vi "关键参数交互.vi"(9 "量程下拉列表":refnum<vi>, 10 "测量模式下拉列表":refnum<vi>, 11 "参数下拉列表":refnum<vi>) -> ()   [LabVIEW 2016, in "斯坦道总磷总氮.lvlib"]
panel:
  out "x != y? 4":T1
  out "x != y? 3":T1
  out "x != y? 2":T1
  out "x != y?":T1
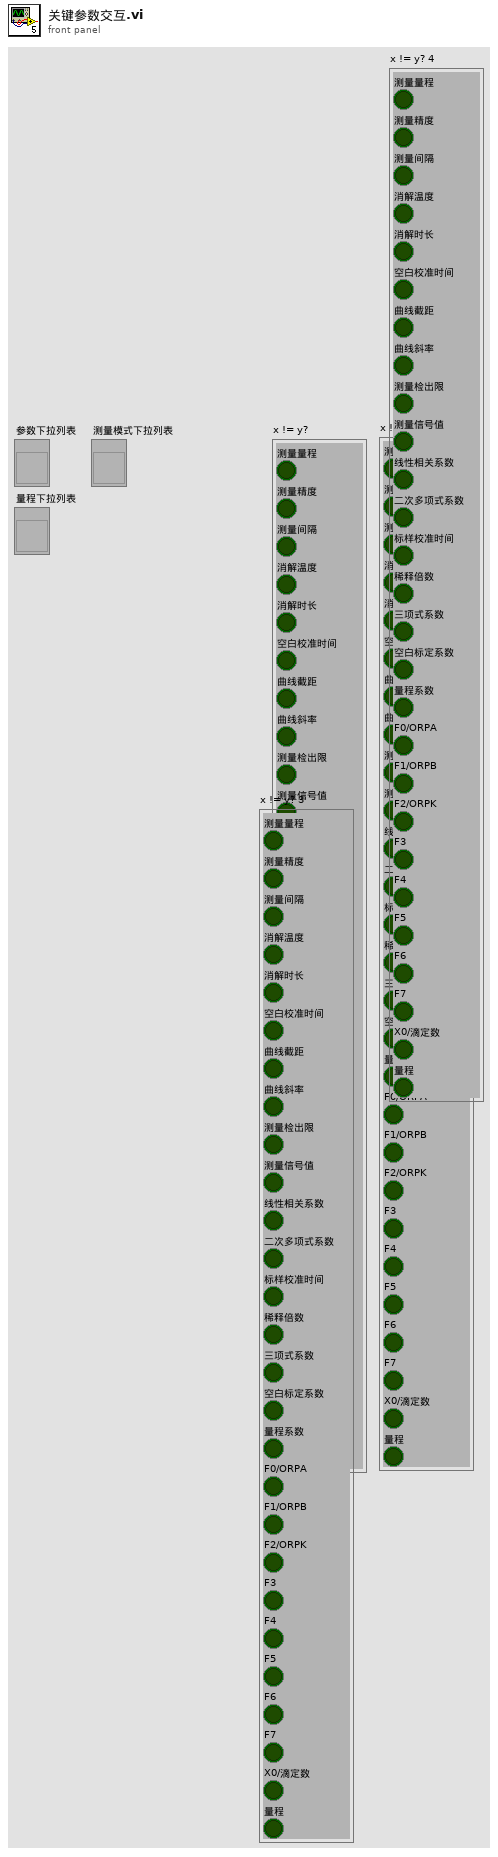
[diagram p1: front panel]
types:
  T1 = cluster{"测量量程":bool, "测量精度":bool, "测量间隔":bool, "消解温度":bool, "消解时长":bool, "空白校准时间":bool, "曲线截距":bool, "曲线斜率":bool, "测量检出限":bool, "测量信号值":bool, "线性相关系数":bool, "二次多项式系数":bool, "标样校准时间":bool, "稀释倍数":bool, "三项式系数":bool, "空白标定系数":bool, "量程系数":bool, "F0/ORPA":bool, "F1/ORPB":bool, "F2/ORPK":bool, "F3":bool, "F4":bool, "F5":bool, "F6":bool, "F7":bool, "X0/滴定数":bool, "量程":bool}
  T2 = cluster{"COD":bool, "氨氮":bool, "总氮":bool, "总磷":bool}
  T3 = cluster{"测量量程":dbl, "测量精度":dbl, "测量间隔":dbl, "消解温度":dbl, "消解时长":dbl, "空白校准时间":timestamp, "曲线截距":dbl, "曲线斜率":dbl, "测量检出限":dbl, "测量信号值":dbl, "线性相关系数":dbl, "二次多项式系数":dbl, "标样校准时间":timestamp, "稀释倍数":dbl, "三项式系数":dbl, "空白标定系数":dbl, "量程系数":dbl, "F0/ORPA":dbl, "F1/ORPB":dbl, "F2/ORPK":dbl, "F3":dbl, "F4":dbl, "F5":dbl, "F6":dbl, "F7":dbl, "X0/滴定数":dbl, "量程":dbl}
  T4 = cluster{"chose":string, "公式":cluster{"X^2":dbl, "X":dbl, "b":dbl}}
  T5 = cluster{"时间标识":timestamp, "设备":string, "日志信息":string, "流程参数":string}
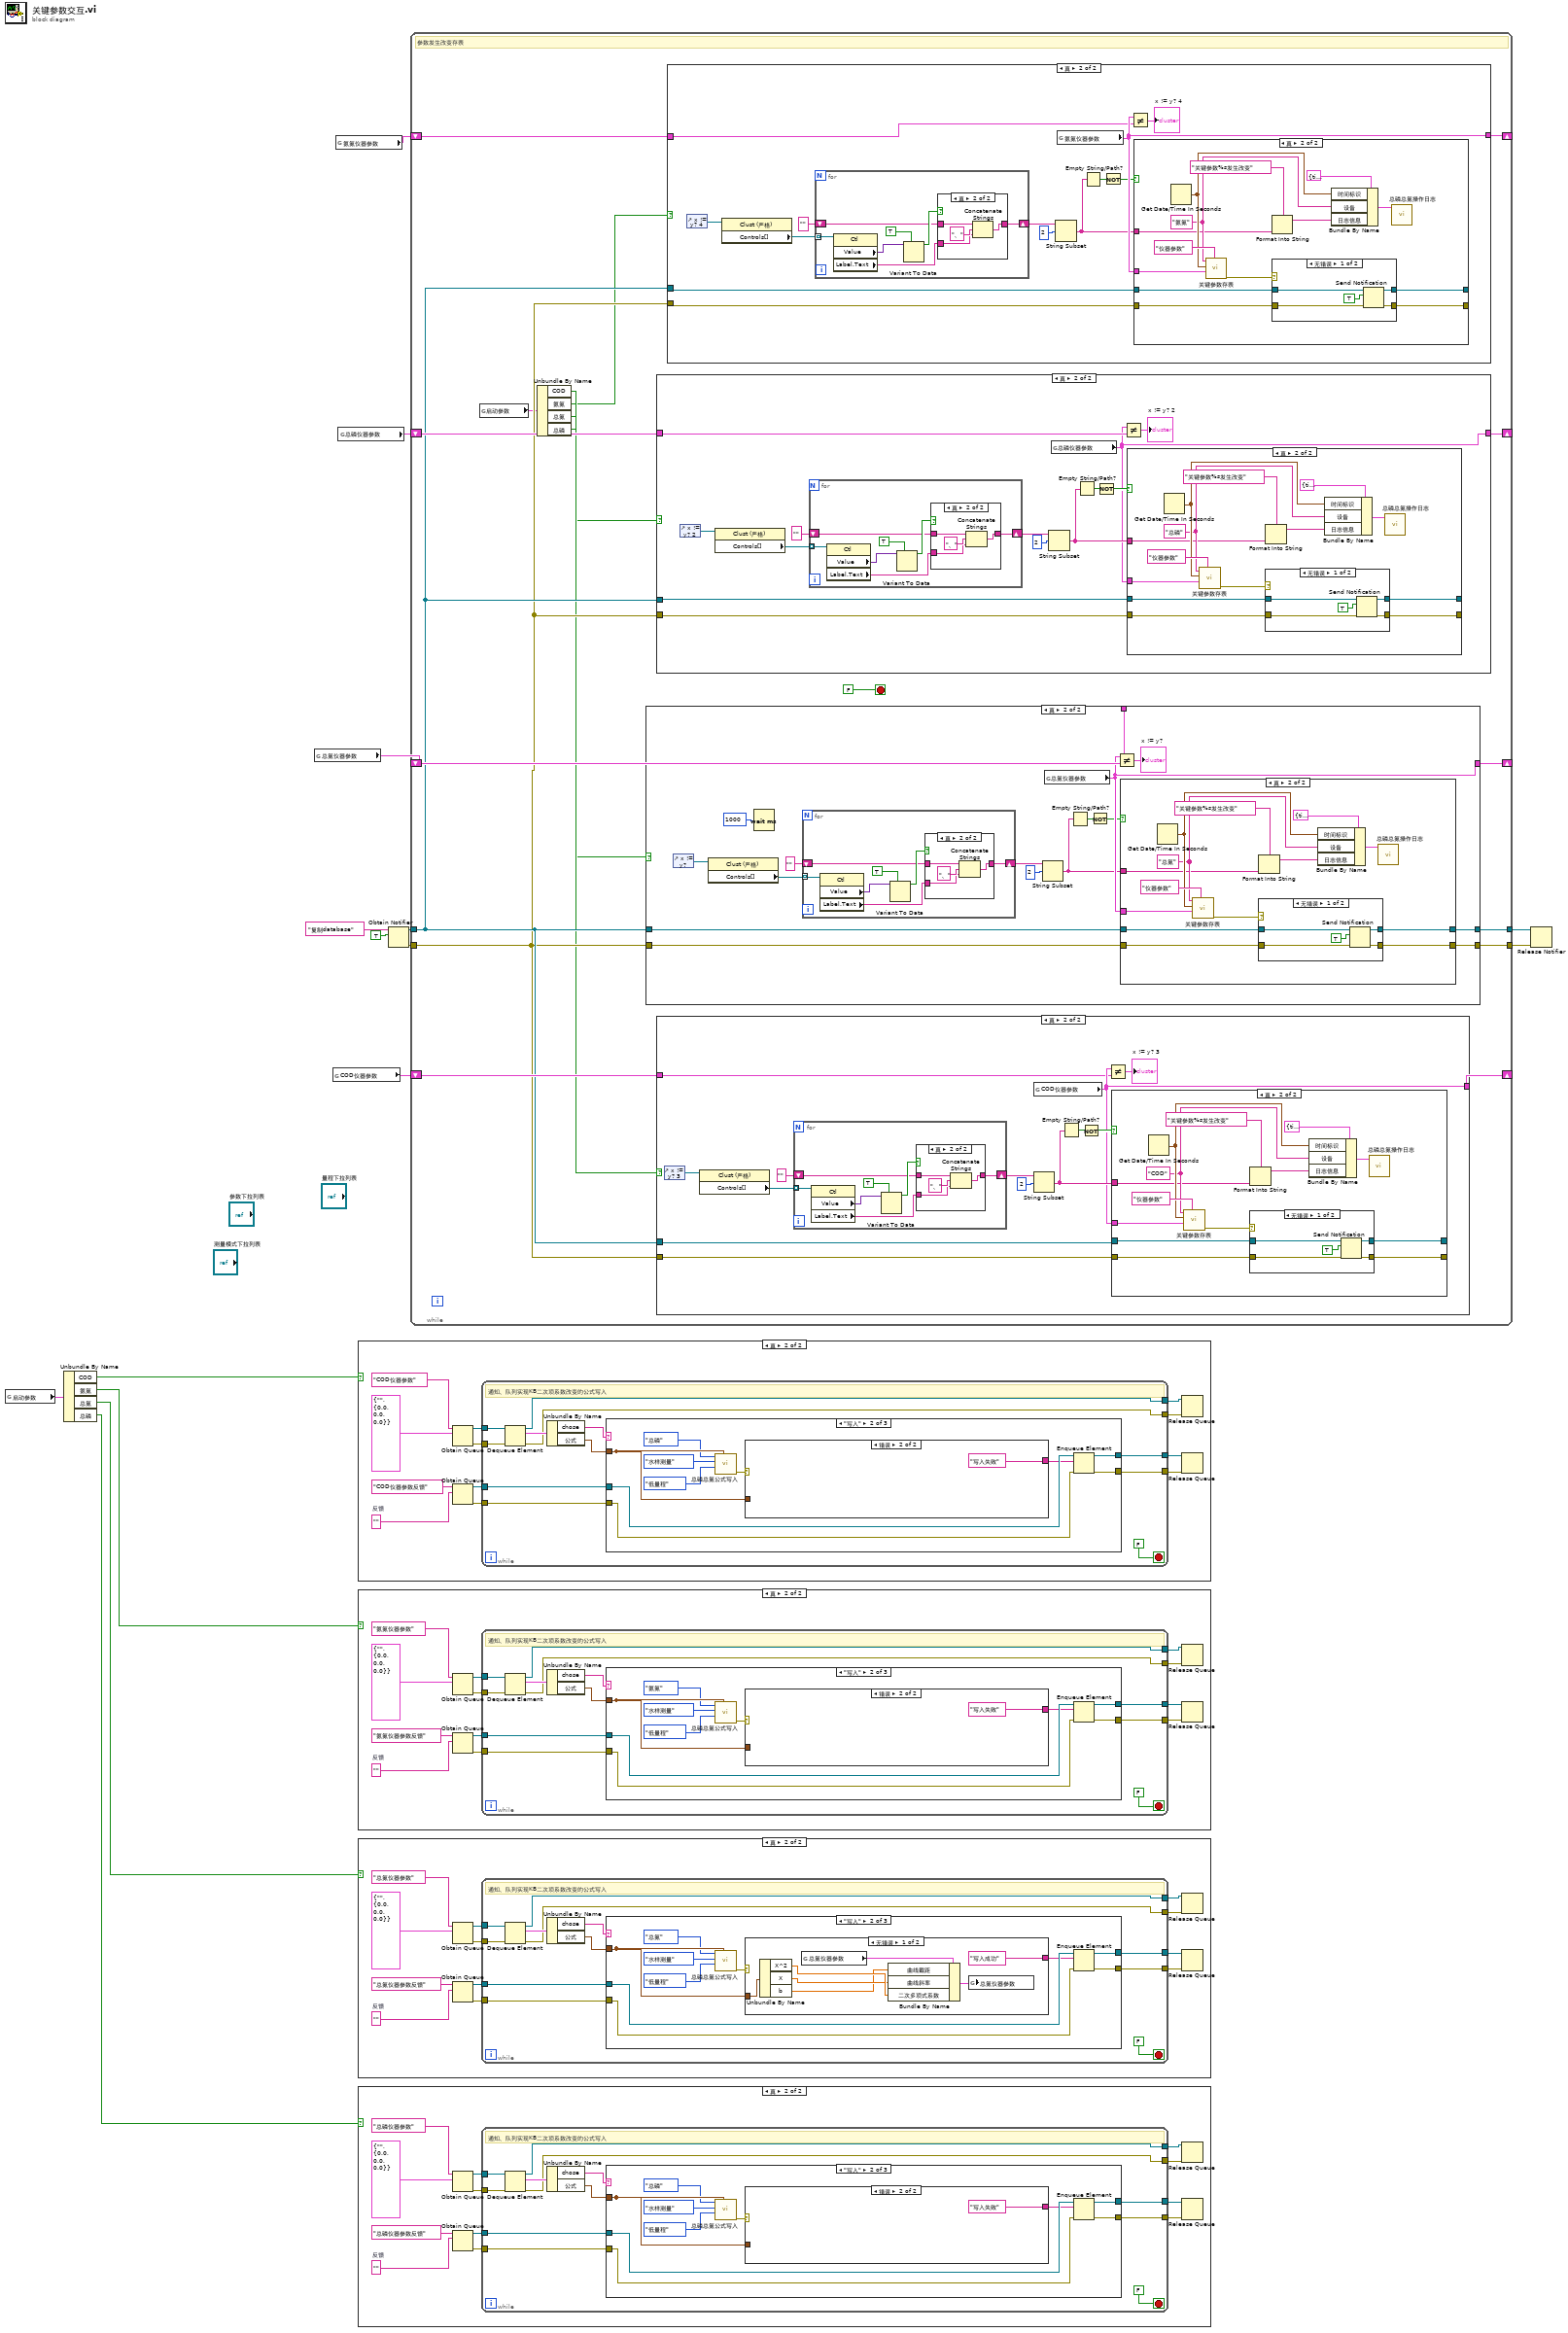
[diagram p0: block diagram]
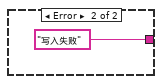
[diagram p4: hidden frame]
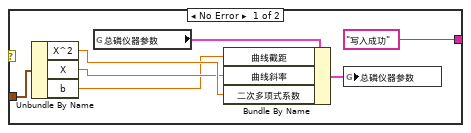
[diagram p8: hidden frame]
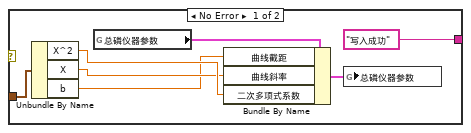
[diagram p12: hidden frame]
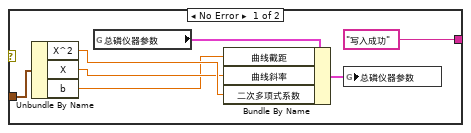
[diagram p16: hidden frame]
diagram:
  n1 = global read "总磷总氮断电保存全局变量.vi" "启动参数"() -> (w6:T2)
  n2 = Unbundle By Name(w6) -> ("COD"=w5:bool, "氨氮"=w4:bool, "总氮"=w2:bool, "总磷"=w3:bool)
  n3 = global read "总磷总氮断电保存全局变量.vi" "总氮仪器参数"() -> (w15:T3)
  n4 = global read "总磷总氮断电保存全局变量.vi" "COD仪器参数"() -> (w7:T3)
  n5 = global read "总磷总氮断电保存全局变量.vi" "氨氮仪器参数"() -> (w1:T3)
  n6 = global read "总磷总氮断电保存全局变量.vi" "总磷仪器参数"() -> (w8:T3)
  n7 = case shown="真" w5 {
    frame False {
    }
    frame True {
      w22 = ""  # 反馈
      n8 = Obtain Queue(name (unnamed)="COD仪器参数" ("名称（未命名）"), element data type=T4 {"chose"="", "公式"={"X^2"=0.0, "X"=0.0, "b"=0.0}}) -> (queue out=w26:refnum<queue>, error out=w27:errorcluster)  [unwired: 3 in, 1 out]
      n9 = Obtain Queue(name (unnamed)="COD仪器参数反馈" ("名称（未命名）"), element data type=w22) -> (queue out=w21:refnum<queue>, error out=w23:errorcluster)  [unwired: 3 in, 1 out]
      n10 = while {
        tunnel: w26 -> [w38]
        tunnel: w27 -> [w37]
        tunnel: [w29] -> w18
        tunnel: [w28] -> w19
        tunnel: w21 -> [w33]
        tunnel: w23 -> [w32]
        tunnel: [w31] -> w24
        tunnel: [w30] -> w25
        stop <- FALSE stop-if-true
        # "通知、队列实现KB二次项系数改变的公式写入"
        n11 = Dequeue Element(queue=w38, error in (no error)=w37) -> (queue out=w29:refnum<queue>, element=w36:T4, error out=w28:errorcluster)  [unwired: 1 in, 1 out]
        n12 = Unbundle By Name(w36) -> ("chose"=w35:string, "公式"=w34:cluster{"X^2":dbl, "X":dbl, "b":dbl})
        n13 = case shown="\"写入\"" w35 {
          tunnel: w34 -> [_ w45 _]
          tunnel: w33 -> [w41 w50 w61]
          tunnel: w32 -> [w40 w48 w60]
          tunnel: [w41 w47 w61] -> w31
          tunnel: [w40 w46 w60] -> w30
          frame "假", Default {
          }
          frame "写入" {
            n14 = call "总磷总氮公式写入.vi"("公式"=w45, "量程"=enum16{"低量程", "高量程"}."低量程", "测量模式"=enum16{"水样测量", "零点核查", "跨度核查", "标样核查", "加标回收"}."水样测量", "测量参数"=enum16{"COD", "氨氮", "总氮", "总磷"}."总磷") -> ("error out"=w51:errorcluster)  [unwired: 7 in]
            n15 = case shown="错误" w51 {
              tunnel: ["写入成功" ("消息") "写入失败" ("消息")] -> w49
              tunnel: w45 -> [w55 _]
              frame No Error {
                n16 = Unbundle By Name(w55) -> ("X^2"=w54:dbl, "X"=w53:dbl, "b"=w52:dbl)
                n17 = global read "总磷总氮断电保存全局变量.vi" "总磷仪器参数"() -> (w56:T3)
                n18 = Bundle By Name(cluster=w56, "曲线截距"=w52, "曲线斜率"=w53, "二次多项式系数"=w54) -> (w57:T3)
                n19 = global write "总磷总氮断电保存全局变量.vi" "总磷仪器参数"(w57) -> ()
              }
              frame Error {
              }
            }
            n20 = Enqueue Element(queue=w50, element=w49, error in (no error)=w48) -> (queue out=w47:refnum<queue>, error out=w46:errorcluster)  [unwired: 1 in, 1 out]
          }
          frame "读取" {
          }
        }
      }
      n21 = Release Queue(queue=w18, error in (no error)=w19) -> ()  [unwired: 1 in, 3 out]
      n22 = Release Queue(queue=w24, error in (no error)=w25) -> ()  [unwired: 1 in, 3 out]
    }
  }
  n23 = case shown="真" w4 {
    frame False {
    }
    frame True {
      w67 = ""  # 反馈
      n24 = Obtain Queue(name (unnamed)="氨氮仪器参数" ("名称（未命名）"), element data type=T4 {"chose"="", "公式"={"X^2"=0.0, "X"=0.0, "b"=0.0}}) -> (queue out=w63:refnum<queue>, error out=w62:errorcluster)  [unwired: 3 in, 1 out]
      n25 = Obtain Queue(name (unnamed)="氨氮仪器参数反馈" ("名称（未命名）"), element data type=w67) -> (queue out=w68:refnum<queue>, error out=w66:errorcluster)  [unwired: 3 in, 1 out]
      n26 = while {
        tunnel: w63 -> [w84]
        tunnel: w62 -> [w83]
        tunnel: [w75] -> w71
        tunnel: [w74] -> w70
        tunnel: w68 -> [w79]
        tunnel: w66 -> [w78]
        tunnel: [w77] -> w65
        tunnel: [w76] -> w64
        stop <- FALSE stop-if-true
        # "通知、队列实现KB二次项系数改变的公式写入"
        n27 = Dequeue Element(queue=w84, error in (no error)=w83) -> (queue out=w75:refnum<queue>, element=w82:T4, error out=w74:errorcluster)  [unwired: 1 in, 1 out]
        n28 = Unbundle By Name(w82) -> ("chose"=w81:string, "公式"=w80:cluster{"X^2":dbl, "X":dbl, "b":dbl})
        n29 = case shown="\"写入\"" w81 {
          tunnel: w80 -> [_ w91 _]
          tunnel: w79 -> [w87 w96 w107]
          tunnel: w78 -> [w86 w94 w106]
          tunnel: [w87 w93 w107] -> w77
          tunnel: [w86 w92 w106] -> w76
          frame "假", Default {
          }
          frame "写入" {
            n30 = call "总磷总氮公式写入.vi"("公式"=w91, "量程"=enum16{"低量程", "高量程"}."低量程", "测量模式"=enum16{"水样测量", "零点核查", "跨度核查", "标样核查", "加标回收"}."水样测量", "测量参数"=enum16{"COD", "氨氮", "总氮", "总磷"}."氨氮") -> ("error out"=w97:errorcluster)  [unwired: 7 in]
            n31 = case shown="错误" w97 {
              tunnel: ["写入成功" ("消息") "写入失败" ("消息")] -> w95
              tunnel: w91 -> [w101 _]
              frame No Error {
                n32 = Unbundle By Name(w101) -> ("X^2"=w100:dbl, "X"=w99:dbl, "b"=w98:dbl)
                n33 = global read "总磷总氮断电保存全局变量.vi" "总磷仪器参数"() -> (w102:T3)
                n34 = Bundle By Name(cluster=w102, "曲线截距"=w98, "曲线斜率"=w99, "二次多项式系数"=w100) -> (w103:T3)
                n35 = global write "总磷总氮断电保存全局变量.vi" "总磷仪器参数"(w103) -> ()
              }
              frame Error {
              }
            }
            n36 = Enqueue Element(queue=w96, element=w95, error in (no error)=w94) -> (queue out=w93:refnum<queue>, error out=w92:errorcluster)  [unwired: 1 in, 1 out]
          }
          frame "读取" {
          }
        }
      }
      n37 = Release Queue(queue=w71, error in (no error)=w70) -> ()  [unwired: 1 in, 3 out]
      n38 = Release Queue(queue=w65, error in (no error)=w64) -> ()  [unwired: 1 in, 3 out]
    }
  }
  n39 = case shown="真" w2 {
    frame False {
    }
    frame True {
      w113 = ""  # 反馈
      n40 = Obtain Queue(name (unnamed)="总氮仪器参数" ("名称（未命名）"), element data type=T4 {"chose"="", "公式"={"X^2"=0.0, "X"=0.0, "b"=0.0}}) -> (queue out=w109:refnum<queue>, error out=w108:errorcluster)  [unwired: 3 in, 1 out]
      n41 = Obtain Queue(name (unnamed)="总氮仪器参数反馈" ("名称（未命名）"), element data type=w113) -> (queue out=w114:refnum<queue>, error out=w112:errorcluster)  [unwired: 3 in, 1 out]
      n42 = while {
        tunnel: w109 -> [w130]
        tunnel: w108 -> [w129]
        tunnel: [w121] -> w117
        tunnel: [w120] -> w116
        tunnel: w114 -> [w125]
        tunnel: w112 -> [w124]
        tunnel: [w123] -> w111
        tunnel: [w122] -> w110
        stop <- FALSE stop-if-true
        # "通知、队列实现KB二次项系数改变的公式写入"
        n43 = Dequeue Element(queue=w130, error in (no error)=w129) -> (queue out=w121:refnum<queue>, element=w128:T4, error out=w120:errorcluster)  [unwired: 1 in, 1 out]
        n44 = Unbundle By Name(w128) -> ("chose"=w127:string, "公式"=w126:cluster{"X^2":dbl, "X":dbl, "b":dbl})
        n45 = case shown="\"写入\"" w127 {
          tunnel: w126 -> [_ w137 _]
          tunnel: w125 -> [w133 w142 w153]
          tunnel: w124 -> [w132 w140 w152]
          tunnel: [w133 w139 w153] -> w123
          tunnel: [w132 w138 w152] -> w122
          frame "假", Default {
          }
          frame "写入" {
            n46 = call "总磷总氮公式写入.vi"("公式"=w137, "量程"=enum16{"低量程", "高量程"}."低量程", "测量模式"=enum16{"水样测量", "零点核查", "跨度核查", "标样核查", "加标回收"}."水样测量", "测量参数"=enum16{"COD", "氨氮", "总氮", "总磷"}."总氮") -> ("error out"=w143:errorcluster)  [unwired: 7 in]
            n47 = case shown="无错误" w143 {
              tunnel: ["写入成功" ("消息") "写入失败" ("消息")] -> w141
              tunnel: w137 -> [w147 _]
              frame No Error {
                n48 = Unbundle By Name(w147) -> ("X^2"=w146:dbl, "X"=w145:dbl, "b"=w144:dbl)
                n49 = global read "总磷总氮断电保存全局变量.vi" "总氮仪器参数"() -> (w148:T3)
                n50 = Bundle By Name(cluster=w148, "曲线截距"=w144, "曲线斜率"=w145, "二次多项式系数"=w146) -> (w149:T3)
                n51 = global write "总磷总氮断电保存全局变量.vi" "总氮仪器参数"(w149) -> ()
              }
              frame Error {
              }
            }
            n52 = Enqueue Element(queue=w142, element=w141, error in (no error)=w140) -> (queue out=w139:refnum<queue>, error out=w138:errorcluster)  [unwired: 1 in, 1 out]
          }
          frame "读取" {
          }
        }
      }
      n53 = Release Queue(queue=w117, error in (no error)=w116) -> ()  [unwired: 1 in, 3 out]
      n54 = Release Queue(queue=w111, error in (no error)=w110) -> ()  [unwired: 1 in, 3 out]
    }
  }
  n55 = case shown="真" w3 {
    frame False {
    }
    frame True {
      w160 = ""  # 反馈
      n56 = Obtain Queue(name (unnamed)="总磷仪器参数" ("名称（未命名）"), element data type=T4 {"chose"="", "公式"={"X^2"=0.0, "X"=0.0, "b"=0.0}}) -> (queue out=w164:refnum<queue>, error out=w165:errorcluster)  [unwired: 3 in, 1 out]
      n57 = Obtain Queue(name (unnamed)="总磷仪器参数反馈" ("名称（未命名）"), element data type=w160) -> (queue out=w159:refnum<queue>, error out=w161:errorcluster)  [unwired: 3 in, 1 out]
      n58 = while {
        tunnel: w164 -> [w176]
        tunnel: w165 -> [w175]
        tunnel: [w167] -> w156
        tunnel: [w166] -> w157
        tunnel: w159 -> [w171]
        tunnel: w161 -> [w170]
        tunnel: [w169] -> w162
        tunnel: [w168] -> w163
        stop <- FALSE stop-if-true
        # "通知、队列实现KB二次项系数改变的公式写入"
        n59 = Dequeue Element(queue=w176, error in (no error)=w175) -> (queue out=w167:refnum<queue>, element=w174:T4, error out=w166:errorcluster)  [unwired: 1 in, 1 out]
        n60 = Unbundle By Name(w174) -> ("chose"=w173:string, "公式"=w172:cluster{"X^2":dbl, "X":dbl, "b":dbl})
        n61 = case shown="\"写入\"" w173 {
          tunnel: w172 -> [_ w183 _]
          tunnel: w171 -> [w179 w188 w199]
          tunnel: w170 -> [w178 w186 w198]
          tunnel: [w179 w185 w199] -> w169
          tunnel: [w178 w184 w198] -> w168
          frame "假", Default {
          }
          frame "写入" {
            n62 = call "总磷总氮公式写入.vi"("公式"=w183, "量程"=enum16{"低量程", "高量程"}."低量程", "测量模式"=enum16{"水样测量", "零点核查", "跨度核查", "标样核查", "加标回收"}."水样测量", "测量参数"=enum16{"COD", "氨氮", "总氮", "总磷"}."总磷") -> ("error out"=w189:errorcluster)  [unwired: 7 in]
            n63 = case shown="错误" w189 {
              tunnel: ["写入成功" ("消息") "写入失败" ("消息")] -> w187
              tunnel: w183 -> [w193 _]
              frame No Error {
                n64 = Unbundle By Name(w193) -> ("X^2"=w192:dbl, "X"=w191:dbl, "b"=w190:dbl)
                n65 = global read "总磷总氮断电保存全局变量.vi" "总磷仪器参数"() -> (w194:T3)
                n66 = Bundle By Name(cluster=w194, "曲线截距"=w190, "曲线斜率"=w191, "二次多项式系数"=w192) -> (w195:T3)
                n67 = global write "总磷总氮断电保存全局变量.vi" "总磷仪器参数"(w195) -> ()
              }
              frame Error {
              }
            }
            n68 = Enqueue Element(queue=w188, element=w187, error in (no error)=w186) -> (queue out=w185:refnum<queue>, error out=w184:errorcluster)  [unwired: 1 in, 1 out]
          }
          frame "读取" {
          }
        }
      }
      n69 = Release Queue(queue=w156, error in (no error)=w157) -> ()  [unwired: 1 in, 3 out]
      n70 = Release Queue(queue=w162, error in (no error)=w163) -> ()  [unwired: 1 in, 3 out]
    }
  }
  n71 = Obtain Notifier(name (unnamed)="复制database" ("名称（未命名）"), notification data type=TRUE) -> (notifier out=w12:refnum<notifier>, error out=w11:errorcluster)  [unwired: 2 in, 1 out]
  n72 = while {
    shift-right: [w216] -> _
    shift-left: w15 -> [w217]
    tunnel: w12 -> [w207]
    tunnel: w11 -> [w206]
    tunnel: [w215] -> w10
    tunnel: [w214] -> w9
    shift-right: [w212] -> _
    shift-left: w8 -> [w213]
    shift-right: [w211] -> _
    shift-left: w7 -> [w210]
    shift-right: [w209] -> _
    shift-left: w1 -> [w208]
    stop <- FALSE stop-if-true
    # "参数发生改变存表"
    n73 = global read "总磷总氮断电保存全局变量.vi" "启动参数"() -> (w204:T2)
    n74 = Unbundle By Name(w204) -> ("COD"=w203:bool, "氨氮"=w200:bool, "总氮"=w202:bool, "总磷"=w201:bool)
    n75 = case shown="真" w202 {
      tunnel: w217 -> [w269 w284]
      tunnel: [w269 w281] -> w216
      tunnel: [w268 w280] -> w215
      tunnel: [w267 w279] -> w214
      tunnel: w207 -> [w268 w271]
      tunnel: w206 -> [w267 w270]
      frame False {
      }
      frame True {
        n76 = control-ref of="x != y?"() -> (w282:refnum<vi>)
        n77 = property class="Clust (严格)"(reference=w282) -> ("Controls[]"=w275:refnum<vi>[])  [unwired: 1 in, 2 out]
        n78 = Wait (ms)(milliseconds to wait=u32 1000 ("等待时间（毫秒）")) -> ()  [unwired: 1 out]
        n79 = for {
          tunnel: w275 -> [w292] mode=indexing
          shift-right: [w286] -> w277
          shift-left: "" -> [w288]
          n80 = property class="Ctl"(reference=w292) -> ("Value"=w290:variant, "Label.Text"=w287:string)  [unwired: 1 in, 2 out]
          n81 = Variant To Data(type=TRUE, Variant=w290) -> (data=w289:bool)  [unwired: 1 in, 1 out]
          n82 = case shown="真" w289 {
            tunnel: w288 -> [w293 w297]
            tunnel: w287 -> [_ w294]
            tunnel: [w293 w296] -> w286
            frame False {
            }
            frame True {
              n83 = Concatenate Strings(w297, "、", w294) -> (w296:string)
            }
          }
        }
        n84 = String Subset(string=w277, offset (0)=2 ("偏移量(0)")) -> (substring=w272:string)  [unwired: 1 in]
        n85 = global read "总磷总氮断电保存全局变量.vi" "总氮仪器参数"() -> (w281:T3)
        n86 = Empty String/Path?(string/path=w272) -> (empty?=w274:bool)
        n87 = Not(x=w274) -> (.not. x?=w273:bool)
        n88 = Not Equal?(x=w281, y=w284) -> (x != y?=→"x != y?":T1)
        n89 = case shown="真" w273 {
          tunnel: w281 -> [_ w312]
          tunnel: w272 -> [_ w306]
          tunnel: w271 -> [w299 w304]
          tunnel: w270 -> [w298 w303]
          tunnel: [w299 w301] -> w280
          tunnel: [w298 w300] -> w279
          frame False {
          }
          frame True {
            w308 = "总氮" ("仪器名称")
            n90 = Get Date/Time In Seconds() -> (seconds since 1Jan1904=w309:timestamp)
            n91 = call "关键参数存表.vi"("table"="仪器参数", "仪器参数"=w312, "datatime"=w309, "仪器名称"=w308) -> ("error out"=w302:errorcluster)  [unwired: 7 in]
            n92 = Format Into String(format string="关键参数%s发生改变" ("格式字符串"), w306) -> (resulting string=w305:string)  [unwired: 2 in, 1 out]
            n93 = case shown="无错误" w302 {
              tunnel: w304 -> [w318 w320]
              tunnel: w303 -> [w317 w319]
              tunnel: [w315 w320] -> w301
              tunnel: [w314 w319] -> w300
              frame No Error {
                n94 = Send Notification(notification=TRUE ("通知"), notifier=w318, error in (no error)=w317) -> (notifier out=w315:refnum<notifier>, error out=w314:errorcluster)
              }
              frame Error {
              }
            }
            n95 = Bundle By Name(cluster=T5 {"时间标识"=timestamp(0 s since 1904-01-01), "设备"="", "日志信息"="", "流程参数"=""} ("data in"), "时间标识"=w309, "设备"=w308, "日志信息"=w305) -> (w310:T5)
            n96 = call "总磷总氮操作日志.vi"("data in"=w310) -> ()  [unwired: 11 in]
          }
        }
      }
    }
    n97 = case shown="真" w201 {
      tunnel: w213 -> [w321 w325]
      tunnel: [w321 w324] -> w212
      tunnel: w207 -> [_ w323]
      tunnel: w206 -> [_ w322]
      frame False {
      }
      frame True {
        n98 = control-ref of="x != y? 2"() -> (w327:refnum<vi>)
        n99 = property class="Clust (严格)"(reference=w327) -> ("Controls[]"=w331:refnum<vi>[])  [unwired: 1 in, 2 out]
        n100 = for {
          tunnel: w331 -> [w341] mode=indexing
          shift-right: [w335] -> w329
          shift-left: "" -> [w337]
          n101 = property class="Ctl"(reference=w341) -> ("Value"=w339:variant, "Label.Text"=w336:string)  [unwired: 1 in, 2 out]
          n102 = Variant To Data(type=TRUE, Variant=w339) -> (data=w338:bool)  [unwired: 1 in, 1 out]
          n103 = case shown="真" w338 {
            tunnel: w337 -> [w342 w346]
            tunnel: w336 -> [_ w343]
            tunnel: [w342 w345] -> w335
            frame False {
            }
            frame True {
              n104 = Concatenate Strings(w346, "、", w343) -> (w345:string)
            }
          }
        }
        n105 = String Subset(string=w329, offset (0)=2 ("偏移量(0)")) -> (substring=w334:string)  [unwired: 1 in]
        n106 = global read "总磷总氮断电保存全局变量.vi" "总磷仪器参数"() -> (w324:T3)
        n107 = Empty String/Path?(string/path=w334) -> (empty?=w332:bool)
        n108 = Not(x=w332) -> (.not. x?=w333:bool)
        n109 = Not Equal?(x=w324, y=w325) -> (x != y?=→"x != y? 2":T1)
        n110 = case shown="真" w333 {
          tunnel: w324 -> [_ w361]
          tunnel: w334 -> [_ w355]
          tunnel: w323 -> [w348 w353]
          tunnel: w322 -> [w347 w352]
          tunnel: [w348 w350] -> _
          tunnel: [w347 w349] -> _
          frame False {
          }
          frame True {
            w357 = "总磷" ("仪器名称")
            n111 = Get Date/Time In Seconds() -> (seconds since 1Jan1904=w358:timestamp)
            n112 = call "关键参数存表.vi"("table"="仪器参数", "仪器参数"=w361, "datatime"=w358, "仪器名称"=w357) -> ("error out"=w351:errorcluster)  [unwired: 7 in]
            n113 = Format Into String(format string="关键参数%s发生改变" ("格式字符串"), w355) -> (resulting string=w354:string)  [unwired: 2 in, 1 out]
            n114 = case shown="无错误" w351 {
              tunnel: w353 -> [w367 w369]
              tunnel: w352 -> [w366 w368]
              tunnel: [w364 w369] -> w350
              tunnel: [w363 w368] -> w349
              frame No Error {
                n115 = Send Notification(notification=TRUE ("通知"), notifier=w367, error in (no error)=w366) -> (notifier out=w364:refnum<notifier>, error out=w363:errorcluster)
              }
              frame Error {
              }
            }
            n116 = Bundle By Name(cluster=T5 {"时间标识"=timestamp(0 s since 1904-01-01), "设备"="", "日志信息"="", "流程参数"=""} ("data in"), "时间标识"=w358, "设备"=w357, "日志信息"=w354) -> (w359:T5)
            n117 = call "总磷总氮操作日志.vi"("data in"=w359) -> ()  [unwired: 11 in]
          }
        }
      }
    }
    n118 = case shown="真" w203 {
      tunnel: [w218 w224] -> w211
      tunnel: w210 -> [w218 w221]
      tunnel: w207 -> [_ w220]
      tunnel: w206 -> [_ w219]
      frame False {
      }
      frame True {
        n119 = control-ref of="x != y? 3"() -> (w223:refnum<vi>)
        n120 = property class="Clust (严格)"(reference=w223) -> ("Controls[]"=w228:refnum<vi>[])  [unwired: 1 in, 2 out]
        n121 = for {
          tunnel: w228 -> [w238] mode=indexing
          shift-right: [w232] -> w226
          shift-left: "" -> [w234]
          n122 = property class="Ctl"(reference=w238) -> ("Value"=w236:variant, "Label.Text"=w233:string)  [unwired: 1 in, 2 out]
          n123 = Variant To Data(type=TRUE, Variant=w236) -> (data=w235:bool)  [unwired: 1 in, 1 out]
          n124 = case shown="真" w235 {
            tunnel: w234 -> [w239 w243]
            tunnel: w233 -> [_ w240]
            tunnel: [w239 w242] -> w232
            frame False {
            }
            frame True {
              n125 = Concatenate Strings(w243, "、", w240) -> (w242:string)
            }
          }
        }
        n126 = String Subset(string=w226, offset (0)=2 ("偏移量(0)")) -> (substring=w231:string)  [unwired: 1 in]
        n127 = global read "总磷总氮断电保存全局变量.vi" "COD仪器参数"() -> (w224:T3)
        n128 = Empty String/Path?(string/path=w231) -> (empty?=w229:bool)
        n129 = Not(x=w229) -> (.not. x?=w230:bool)
        n130 = Not Equal?(x=w224, y=w221) -> (x != y?=→"x != y? 3":T1)
        n131 = case shown="真" w230 {
          tunnel: w224 -> [_ w258]
          tunnel: w231 -> [_ w252]
          tunnel: w220 -> [w245 w250]
          tunnel: w219 -> [w244 w249]
          tunnel: [w245 w247] -> _
          tunnel: [w244 w246] -> _
          frame False {
          }
          frame True {
            w254 = "COD" ("仪器名称")
            n132 = Get Date/Time In Seconds() -> (seconds since 1Jan1904=w255:timestamp)
            n133 = call "关键参数存表.vi"("table"="仪器参数", "仪器参数"=w258, "datatime"=w255, "仪器名称"=w254) -> ("error out"=w248:errorcluster)  [unwired: 7 in]
            n134 = Format Into String(format string="关键参数%s发生改变" ("格式字符串"), w252) -> (resulting string=w251:string)  [unwired: 2 in, 1 out]
            n135 = case shown="无错误" w248 {
              tunnel: w250 -> [w264 w266]
              tunnel: w249 -> [w263 w265]
              tunnel: [w261 w266] -> w247
              tunnel: [w260 w265] -> w246
              frame No Error {
                n136 = Send Notification(notification=TRUE ("通知"), notifier=w264, error in (no error)=w263) -> (notifier out=w261:refnum<notifier>, error out=w260:errorcluster)
              }
              frame Error {
              }
            }
            n137 = Bundle By Name(cluster=T5 {"时间标识"=timestamp(0 s since 1904-01-01), "设备"="", "日志信息"="", "流程参数"=""} ("data in"), "时间标识"=w255, "设备"=w254, "日志信息"=w251) -> (w256:T5)
            n138 = call "总磷总氮操作日志.vi"("data in"=w256) -> ()  [unwired: 11 in]
          }
        }
      }
    }
    n139 = case shown="真" w200 {
      tunnel: [w370 w383] -> w209
      tunnel: w208 -> [w370 w382]
      tunnel: w207 -> [_ w372]
      tunnel: w206 -> [_ w371]
      frame False {
      }
      frame True {
        n140 = control-ref of="x != y? 4"() -> (w380:refnum<vi>)
        n141 = property class="Clust (严格)"(reference=w380) -> ("Controls[]"=w376:refnum<vi>[])  [unwired: 1 in, 2 out]
        n142 = for {
          tunnel: w376 -> [w390] mode=indexing
          shift-right: [w384] -> w378
          shift-left: "" -> [w386]
          n143 = property class="Ctl"(reference=w390) -> ("Value"=w388:variant, "Label.Text"=w385:string)  [unwired: 1 in, 2 out]
          n144 = Variant To Data(type=TRUE, Variant=w388) -> (data=w387:bool)  [unwired: 1 in, 1 out]
          n145 = case shown="真" w387 {
            tunnel: w386 -> [w391 w395]
            tunnel: w385 -> [_ w392]
            tunnel: [w391 w394] -> w384
            frame False {
            }
            frame True {
              n146 = Concatenate Strings(w395, "、", w392) -> (w394:string)
            }
          }
        }
        n147 = String Subset(string=w378, offset (0)=2 ("偏移量(0)")) -> (substring=w373:string)  [unwired: 1 in]
        n148 = global read "总磷总氮断电保存全局变量.vi" "氨氮仪器参数"() -> (w383:T3)
        n149 = Empty String/Path?(string/path=w373) -> (empty?=w375:bool)
        n150 = Not(x=w375) -> (.not. x?=w374:bool)
        n151 = Not Equal?(x=w383, y=w382) -> (x != y?=→"x != y? 4":T1)
        n152 = case shown="真" w374 {
          tunnel: w383 -> [_ w410]
          tunnel: w373 -> [_ w404]
          tunnel: w372 -> [w397 w402]
          tunnel: w371 -> [w396 w401]
          tunnel: [w397 w399] -> _
          tunnel: [w396 w398] -> _
          frame False {
          }
          frame True {
            w406 = "氨氮" ("仪器名称")
            n153 = Get Date/Time In Seconds() -> (seconds since 1Jan1904=w407:timestamp)
            n154 = call "关键参数存表.vi"("table"="仪器参数", "仪器参数"=w410, "datatime"=w407, "仪器名称"=w406) -> ("error out"=w400:errorcluster)  [unwired: 7 in]
            n155 = Format Into String(format string="关键参数%s发生改变" ("格式字符串"), w404) -> (resulting string=w403:string)  [unwired: 2 in, 1 out]
            n156 = case shown="无错误" w400 {
              tunnel: w402 -> [w416 w418]
              tunnel: w401 -> [w415 w417]
              tunnel: [w413 w418] -> w399
              tunnel: [w412 w417] -> w398
              frame No Error {
                n157 = Send Notification(notification=TRUE ("通知"), notifier=w416, error in (no error)=w415) -> (notifier out=w413:refnum<notifier>, error out=w412:errorcluster)
              }
              frame Error {
              }
            }
            n158 = Bundle By Name(cluster=T5 {"时间标识"=timestamp(0 s since 1904-01-01), "设备"="", "日志信息"="", "流程参数"=""} ("data in"), "时间标识"=w407, "设备"=w406, "日志信息"=w403) -> (w408:T5)
            n159 = call "总磷总氮操作日志.vi"("data in"=w408) -> ()  [unwired: 11 in]
          }
        }
      }
    }
  }
  n160 = Release Notifier(notifier=w10, error in (no error)=w9) -> ()  [unwired: 1 in, 3 out]
